vi "Build Concrete Do.vi"(4 "Abstract class path":path, 5 "Target":refnum<vi>, 6 "Class Name":string, 7 "AppInst":refnum<vi>, 8 "error in (no error)":errorcluster, 9 "Actor class path":path, 10 "Do Method path":path, 11 "Target Actor Method path":path) -> (0 "error out":errorcluster)   [LabVIEW 2020, in "Message Maker.lvlib"]
uses:
  Message Maker.lvlib
  <vilib>/Utility/traverseref.llb/TRef TravTarget.ctl
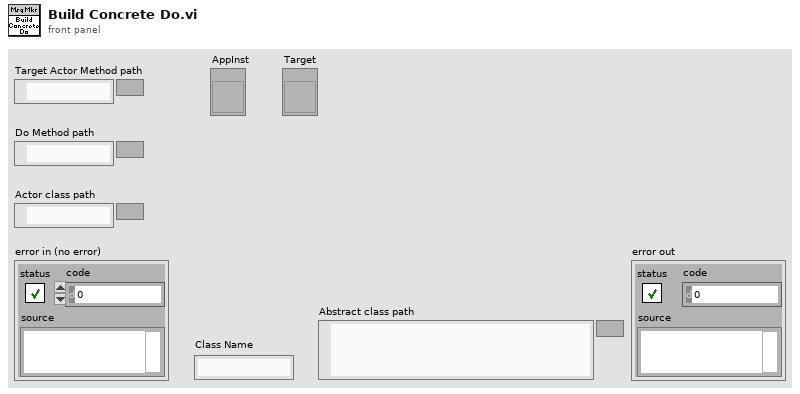
[diagram p1: front panel]
types:
  T1 = enum32{"Invalid", "Standard", "Closed", "Hidden", "Minimized", "Maximized"}
  T2 = typedef "TRef TravTarget.ctl" = enum16{"FP", "BD", "Other"}
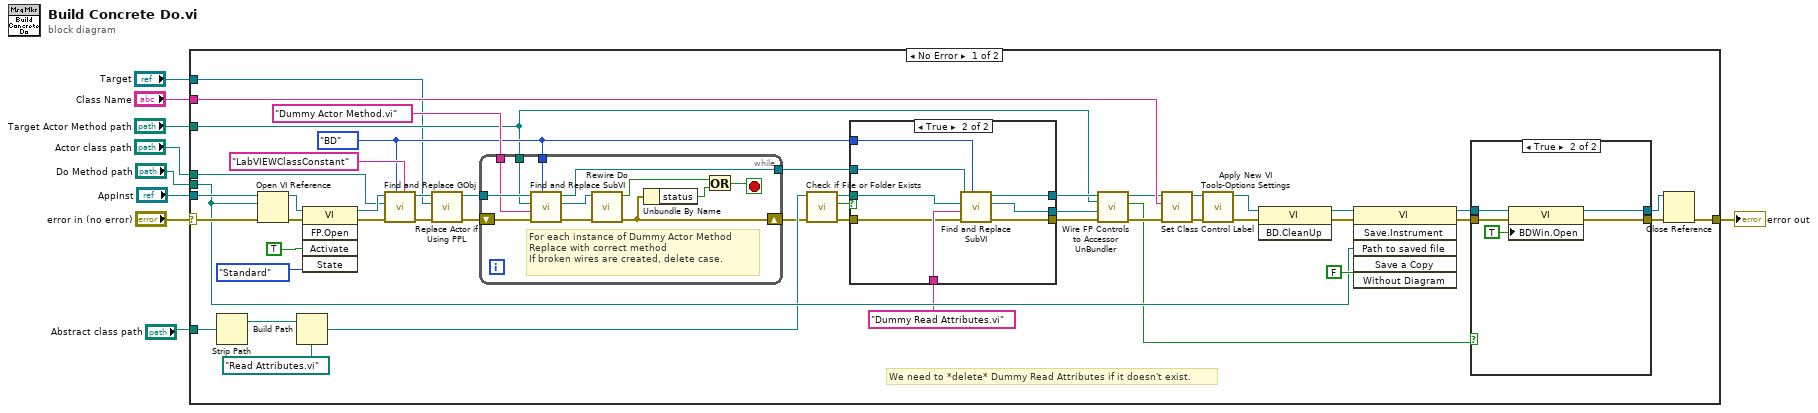
[diagram p0: block diagram]
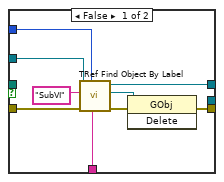
[diagram p2: hidden frame]
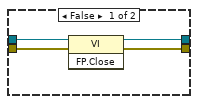
[diagram p3: hidden frame]
diagram:
  n1 = case shown="No Error" "error in (no error)" {
    selector: "error in (no error)" -> [w45 w96]
    tunnel: [w55 w96] -> w2
    tunnel: "Target Actor Method path" -> [w13 _]
    tunnel: "Do Method path" -> [w38 _]
    tunnel: "Actor class path" -> [w46 _]
    tunnel: "Class Name" -> [w44 _]
    tunnel: "AppInst" -> [w39 _]
    tunnel: "Abstract class path" -> [w31 _]
    tunnel: "Target" -> [w10 _]
    frame No Error {
      w18 = TRef_TravTarget."BD" ("Traverse Target")
      # "We need to *delete* Dummy Read Attributes if it doesn't exist."
      n2 = Strip Path(path=w31) -> (stripped path=w30:path)  [unwired: 1 out]
      n3 = Open VI Reference(application reference (local)=w39, vi path=w38, error in (no error)=w45) -> (vi reference=w41:refnum<vi>, error out=w40:errorcluster)  [unwired: 3 in]
      n4 = Build Path(base path=w30, name or relative path=path "Read Attributes.vi") -> (appended path=w23:path)
      n5 = invoke class="VI" method="FP.Open"(reference=w41, error in=w40, "Activate"=TRUE ("Activate?"), "State"=T1."Standard") -> (reference out=w51:refnum<vi>, error out=w52:errorcluster)  [unwired: 1 in, 3 out]
      n6 = call "Find and Replace GObj.vi"("GObj Class Name"="LabVIEWClassConstant" ("Class Name"), "Traverse Target"=w18, "error in (no error)"=w52, "Class Path"=w46, "vi reference in"=w51) -> ("error out"=w27:errorcluster, "vi reference out"=w24:refnum<vi>)  [unwired: 4 in, 1 out]
      n7 = call "Replace Actor if Using PPL.vi"("error in (no error)"=w27, "Target"=w10, "Send VI ref in"=w24) -> ("error out"=w26:errorcluster, "Send VI ref out"=w25:refnum<vi>)  [unwired: 7 in]
      n8 = while {
        tunnel: w25 -> [w95]
        tunnel: w13 -> [w93]
        tunnel: w18 -> [w92]
        tunnel: "Dummy Actor Method.vi" ("GObj Class Name") -> [w84]
        tunnel: [w90] -> w33
        shift-right: [w88] -> w21
        shift-left: w26 -> [w94]
        stop <- w85 stop-if-true
        # "For each instance of Dummy Actor Method\nReplace with correct method\nIf broken wires are created, delete case."
        n9 = call "Find and Replace SubVI.vi"("Traverse Target"=w92, "error in (no error)"=w94, "Old VI Name"=w84, "New VI Path"=w93, "vi reference in"=w95) -> ("error out"=w91:errorcluster, "Replace"=w89:refnum<vi>, "vi reference out"=w90:refnum<vi>)  [unwired: 4 in]
        n10 = call "Rewire Do.vi"("error in (no error)"=w91, "Replace"=w89) -> ("error out"=w88:errorcluster, "done?"=w86:bool)  [unwired: 8 in]
        n11 = Unbundle By Name(w88) -> ("status"=w87:bool)
        n12 = Or(x=w86, y=w87) -> (x .or. y?=w85:bool)
      }
      n13 = call <vilib>:"Check if File or Folder Exists.vi"("error in (no error)"=w21, "path"=w23) -> ("error out"=w22:errorcluster, "file or folder exists?"=w19:bool, "dup path"=w20:path)  [unwired: 7 in]
      n14 = case shown="True" w19 {
        tunnel: [w60 w68] -> w17
        tunnel: [w59 w69] -> w16
        tunnel: w33 -> [w65 w74]
        tunnel: "Dummy Read Attributes.vi" ("GObj Class Name") -> [w63 w73]
        tunnel: w18 -> [w58 w72]
        tunnel: w22 -> [w66 w71]
        tunnel: w20 -> [_ w70]
        tunnel: [_ w67] -> w12
        frame False {
          n15 = call <vilib>:"TRef Find Object By Label.vi"("Label"=w63, "Traverse Target"=w58, "error in (no error)"=w66, "Class Name"="SubVI" ("GObj Class Name"), "VI Ref"=w65) -> ("error out"=w61:errorcluster, "Found Obj Ref"=w62:refnum<vi>, "dup VI Ref"=w59:refnum<vi>)  [unwired: 3 in, 1 out]
          n16 = invoke class="GObj" method="Delete"(reference=w62, error in=w61) -> (error out=w60:errorcluster)  [unwired: 1 in, 2 out]
        }
        frame True {
          n17 = call "Find and Replace SubVI.vi"("Traverse Target"=w72, "error in (no error)"=w71, "Old VI Name"=w73, "New VI Path"=w70, "vi reference in"=w74) -> ("error out"=w68:errorcluster, "Replace"=w67:refnum<vi>, "vi reference out"=w69:refnum<vi>)  [unwired: 4 in]
        }
      }
      n18 = call "Wire FP Controls to Accessor UnBundler.vi"("error in (no error)"=w17, "Attribute VI"=w12, "Target Actor Method Path"=w13, "vi reference in"=w16) -> ("error out"=w15:errorcluster, "Open Block Diagram?"=w11:bool, "vi reference out"=w14:refnum<vi>)  [unwired: 5 in]
      n19 = call "Set Class Control Label.vi"("error in (no error)"=w15, "Class Name"=w44, "vi reference in"=w14) -> ("error out"=w34:errorcluster, "vi reference out"=w37:refnum<vi>)  [unwired: 7 in]
      n20 = call <vilib>:"Apply New VI Tools-Options Settings.vi"("error in (no error)"=w34, "VI Refnum"=w37) -> ("error out"=w35:errorcluster, "dup VI Refnum"=w36:refnum<vi>)  [unwired: 8 in]
      n21 = invoke class="VI" method="BD.CleanUp"(reference=w36, error in=w35) -> (reference out=w28:refnum<vi>, error out=w42:errorcluster)  [unwired: 1 in, 1 out]
      n22 = invoke class="VI" method="Save.Instrument"(reference=w28, error in=w42, "Path to saved file"=w38, "Save a Copy"=FALSE) -> (reference out=w49:refnum<vi>, error out=w50:errorcluster)  [unwired: 2 in, 4 out]
      n23 = case shown="True" w11 {
        tunnel: w50 -> [w78 w81]
        tunnel: w49 -> [w77 w83]
        tunnel: [w76 w79] -> w48
        tunnel: [w75 w82] -> w47
        frame False {
          n24 = invoke class="VI" method="FP.Close"(reference=w77, error in=w78) -> (reference out=w75:refnum<vi>, error out=w76:errorcluster)  [unwired: 1 in, 1 out]
        }
        frame True {
          n25 = property class="VI"(reference=w83, error in=w81, "BDWin.Open"=TRUE ("Block Diagram Window:Open")) -> (reference out=w82:refnum<vi>, error out=w79:errorcluster)
        }
      }
      n26 = Close Reference(reference=w47, error in (no error)=w48) -> (error out=w55:errorcluster)
    }
    frame Error {
    }
  }
  "error out" <- w2
